vi "six legs blue.vi"   [LabVIEW 2010, in "Bluetooth.lvrbt"]
uses:
  Bluetooth.lvrbt
  <vilib>/NXT/Block Support/NXT_InputPort.ctl
  <vilib>/NXT/Block Support/NXT_MessageMailbox.ctl
  <vilib>/NXT/Subs/MotorOutput.ctl
  <vilib>/NXT/Dual Mode Library/Display/drawNumber.vi
  <vilib>/NXT/Dual Mode Library/Sensors/Sonar_cm.vi
  <vilib>/NXT/Dual Mode Library/Motors/ResetMotor.vi
types:
  T1 = typedef "NXT_MessageMailbox.ctl" = u8
  T2 = typedef "NXT_InputPort.ctl" = u8
  T3 = typedef "LVHSConnector.ctl" = cluster{"Hardware":string, "Flattened String":string}
  T4 = typedef "MotorOutput.ctl" = u8
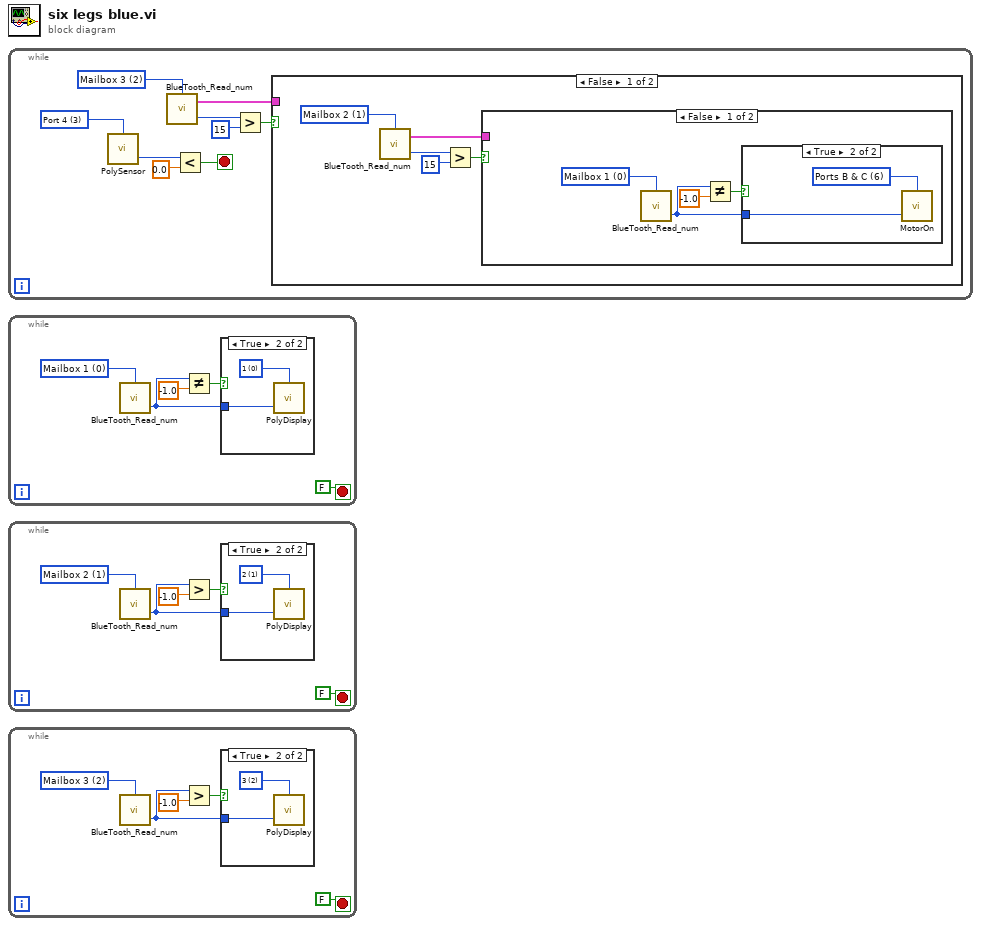
[diagram p0: block diagram]
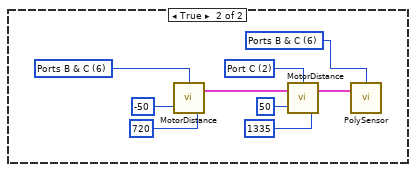
[diagram p6: hidden frame]
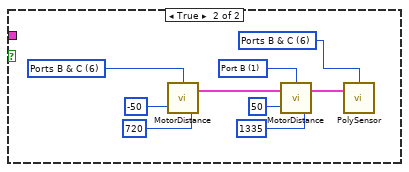
[diagram p7: hidden frame]
diagram:
  n1 = while {
    stop <- w7 stop-if-true
    w1 = T1 2 items=["Mailbox 1", "Mailbox 2", "Mailbox 3", "Mailbox 4", "Mailbox 5", "Mailbox 6", "Mailbox 7", "Mailbox 8", "Mailbox 9", "Mailbox 10"] ("Mailbox")
    w6 = T2 3 items=["Port 1", "Port 2", "Port 3", "Port 4"] ("Port (Port 4)")
    n2 = call-poly <vilib>:"PolySensor.vi"("Port (Port 4)"=w6) -> ("Distance (cm)"=w8:i16)  [unwired: 2 in, 1 out]
    n3 = call <vilib>:"BlueTooth_Read_num.vi"("Mailbox"=w1) -> ("Message"=w4:i32, "NXT"=w5:T3)  [unwired: 2 in]
    n4 = Less?(x=w8, y=0.0) -> (x < y?=w7:bool)
    n5 = Greater?(x=w4, y=15) -> (0:w2:bool)
    n6 = case shown="False" w2 {
      tunnel: w5 -> [_ _]
      frame False {
        w10 = T1 1 items=["Mailbox 1", "Mailbox 2", "Mailbox 3", "Mailbox 4", "Mailbox 5", "Mailbox 6", "Mailbox 7", "Mailbox 8", "Mailbox 9", "Mailbox 10"] ("Mailbox")
        n7 = call <vilib>:"BlueTooth_Read_num.vi"("Mailbox"=w10) -> ("Message"=w14:i32, "NXT"=w11:T3)  [unwired: 2 in]
        n8 = Greater?(x=w14, y=15) -> (0:w12:bool)
        n9 = case shown="False" w12 {
          tunnel: w11 -> [_ _]
          frame False {
            w18 = T1 0 items=["Mailbox 1", "Mailbox 2", "Mailbox 3", "Mailbox 4", "Mailbox 5", "Mailbox 6", "Mailbox 7", "Mailbox 8", "Mailbox 9", "Mailbox 10"] ("Mailbox")
            n10 = call <vilib>:"BlueTooth_Read_num.vi"("Mailbox"=w18) -> ("Message"=w15:i32)  [unwired: 2 in, 1 out]
            n11 = Not Equal?(x=w15, y=-1.0) -> (x != y?=w16:bool)
            n12 = case shown="True" w16 {
              tunnel: w15 -> [_ w19]
              frame False {
              }
              frame True {
                w20 = T4 6 items=["Port A"=0, "Port B"=1, "Port C"=2, "Ports A & B"=4, "Ports A & C"=5, "Ports B & C"=6, "All Ports"=3] ("Output Port (All Ports)")
                n13 = call <vilib>:"MotorOn.vi"("Power (75)"=w19, "Output Port (All Ports)"=w20) -> ()  [unwired: 2 in, 1 out]
              }
            }
          }
          frame True {
            w24 = T4 2 items=["Port A"=0, "Port B"=1, "Port C"=2, "Ports A & B"=4, "Ports A & C"=5, "Ports B & C"=6, "All Ports"=3] ("Output Port (All Ports)")
            w28 = T4 6 items=["Port A"=0, "Port B"=1, "Port C"=2, "Ports A & B"=4, "Ports A & C"=5, "Ports B & C"=6, "All Ports"=3] ("Output Port (All Ports)")
            w21 = T4 6 items=["Port A"=0, "Port B"=1, "Port C"=2, "Ports A & B"=4, "Ports A & C"=5, "Ports B & C"=6, "All Ports"=3] ("Port (All Ports)")
            n14 = call <vilib>:"MotorDistance.vi"("Power (75)"=-50, "Angle of Rotation (360)"=720, "Output Port (All Ports)"=w28) -> ("NXT"=w23:T3)  [unwired: 1 in]
            n15 = call <vilib>:"MotorDistance.vi"("Power (75)"=50, "Angle of Rotation (360)"=1335, "NXT"=w23, "Output Port (All Ports)"=w24) -> ("NXT"=w22:T3)
            n16 = call-poly <vilib>:"PolySensor.vi"("NXT"=w22, "Port (All Ports)"=w21) -> ()  [unwired: 2 in, 1 out]
          }
        }
      }
      frame True {
        w32 = T4 1 items=["Port A"=0, "Port B"=1, "Port C"=2, "Ports A & B"=4, "Ports A & C"=5, "Ports B & C"=6, "All Ports"=3] ("Output Port (All Ports)")
        w36 = T4 6 items=["Port A"=0, "Port B"=1, "Port C"=2, "Ports A & B"=4, "Ports A & C"=5, "Ports B & C"=6, "All Ports"=3] ("Output Port (All Ports)")
        w38 = T4 6 items=["Port A"=0, "Port B"=1, "Port C"=2, "Ports A & B"=4, "Ports A & C"=5, "Ports B & C"=6, "All Ports"=3] ("Port (All Ports)")
        n17 = call <vilib>:"MotorDistance.vi"("Power (75)"=-50, "Angle of Rotation (360)"=720, "Output Port (All Ports)"=w36) -> ("NXT"=w31:T3)  [unwired: 1 in]
        n18 = call <vilib>:"MotorDistance.vi"("Power (75)"=50, "Angle of Rotation (360)"=1335, "NXT"=w31, "Output Port (All Ports)"=w32) -> ("NXT"=w30:T3)
        n19 = call-poly <vilib>:"PolySensor.vi"("NXT"=w30, "Port (All Ports)"=w38) -> ()  [unwired: 2 in, 1 out]
      }
    }
  }
  n20 = while {
    stop <- FALSE stop-if-true
    w42 = T1 0 items=["Mailbox 1", "Mailbox 2", "Mailbox 3", "Mailbox 4", "Mailbox 5", "Mailbox 6", "Mailbox 7", "Mailbox 8", "Mailbox 9", "Mailbox 10"] ("Mailbox")
    n21 = call <vilib>:"BlueTooth_Read_num.vi"("Mailbox"=w42) -> ("Message"=w39:i32)  [unwired: 2 in, 1 out]
    n22 = Not Equal?(x=w39, y=-1.0) -> (x != y?=w40:bool)
    n23 = case shown="True" w40 {
      tunnel: w39 -> [_ w44]
      frame False {
      }
      frame True {
        w45 = i16 0 items=["1", "2", "3", "4", "5", "6", "7", "8"] ("Line")
        n24 = call-poly <vilib>:"PolyDisplay.vi"("number"=w44, "Line"=w45) -> ()  [unwired: 2 in, 1 out]
      }
    }
  }
  n25 = while {
    stop <- FALSE stop-if-true
    w49 = T1 1 items=["Mailbox 1", "Mailbox 2", "Mailbox 3", "Mailbox 4", "Mailbox 5", "Mailbox 6", "Mailbox 7", "Mailbox 8", "Mailbox 9", "Mailbox 10"] ("Mailbox")
    n26 = call <vilib>:"BlueTooth_Read_num.vi"("Mailbox"=w49) -> ("Message"=w46:i32)  [unwired: 2 in, 1 out]
    n27 = Greater?(x=w46, y=-1.0) -> (0:w47:bool)
    n28 = case shown="True" w47 {
      tunnel: w46 -> [_ w51]
      frame False {
      }
      frame True {
        w52 = i16 1 items=["1", "2", "3", "4", "5", "6", "7", "8"] ("Line")
        n29 = call-poly <vilib>:"PolyDisplay.vi"("number"=w51, "Line"=w52) -> ()  [unwired: 2 in, 1 out]
      }
    }
  }
  n30 = while {
    stop <- FALSE stop-if-true
    w56 = T1 2 items=["Mailbox 1", "Mailbox 2", "Mailbox 3", "Mailbox 4", "Mailbox 5", "Mailbox 6", "Mailbox 7", "Mailbox 8", "Mailbox 9", "Mailbox 10"] ("Mailbox")
    n31 = call <vilib>:"BlueTooth_Read_num.vi"("Mailbox"=w56) -> ("Message"=w53:i32)  [unwired: 2 in, 1 out]
    n32 = Greater?(x=w53, y=-1.0) -> (0:w54:bool)
    n33 = case shown="True" w54 {
      tunnel: w53 -> [_ w58]
      frame False {
      }
      frame True {
        w59 = i16 2 items=["1", "2", "3", "4", "5", "6", "7", "8"] ("Line")
        n34 = call-poly <vilib>:"PolyDisplay.vi"("number"=w58, "Line"=w59) -> ()  [unwired: 2 in, 1 out]
      }
    }
  }
